vi "Robot Main.vi"() -> ()   [LabVIEW 2011]
doc: "This VI imlements the framework and scheduler for your robotics program. It should not be necessary to modify the framework. You are expected to add your code to the VIs called from Robot Main, the ones located in the Team Code within the project."
uses:
  GLOBALShooter.vi
panel:
  out "Timings":cluster{"Call Name":string, "Delta (ms)":u32}[](array[cluster])
  in  "Finish":bool
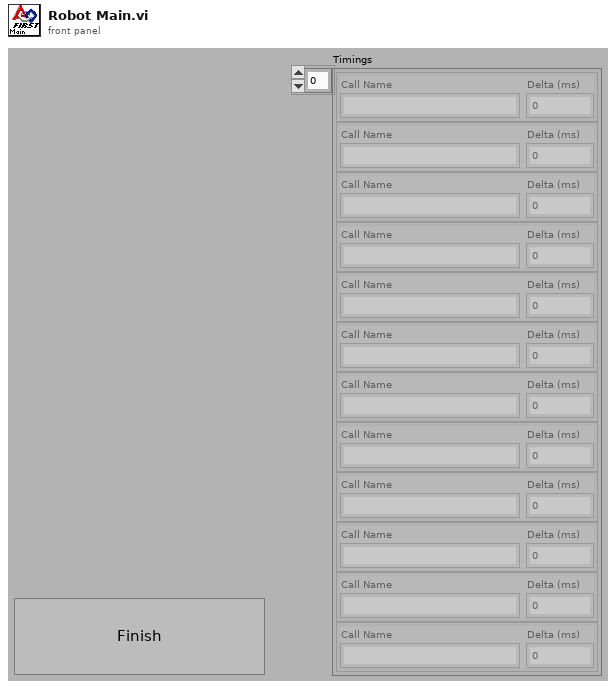
[diagram p1: front panel]
types:
  T1 = typedef "WPI_DriverStationMatch Info.ctl" = cluster{"Autonomous Elapsed Seconds":dbl, "TeleOp Elapsed Seconds":dbl, "Disabled Elapsed Seconds":dbl, "Visited Autonomous":bool, "Visited TeleOp":bool, "Visited Disabled":bool, "Autonomous Settings":cluster{"Autonomous Style":enum16{"Iterative", "Independent"}, "VI Refnum":refnum<vi>}}
  T2 = typedef "WPI_DriverStationDerivedRobotMode.ctl" = enum16{"Init", "Execute", "Stop"}
  T3 = typedef "WPI_DriverStationRobotMode.ctl" = enum16{"Autonomous Disabled", "Autonomous Enabled", "Teleop Disabled", "Teleop Enabled", "Timeout", "Finish"}
  T4 = typedef "WPI_GyroDevRef.ctl" = cluster{"DevStatus":errorcluster, "Analog Module":T5, "Analog Channel":T6, "Offset":dbl, "Gain (VoltsPerDegree/Second)":dbl}
  T5 = typedef "FPGA_TypedefAnalogModule.ctl" = enum16{"Analog Module 1", "Analog Module 2"}
  T6 = typedef "FPGA_AIChannel.ctl" = enum8{"AI 1", "AI 2", "AI 3", "AI 4", "AI 5", "AI 6", "AI 7", "AI 8", "Invalid"}
  T7 = typedef "WPI_EncoderDevRef.ctl" = cluster{"DevStatus":errorcluster, "EncoderIndex":T8, "CounterIndex":T9, "DistancePerCount":dbl, "Decoding Type":T10}
  T8 = typedef "FPGA_EncoderIdx.ctl" = enum8{"Enc 0", "Enc 1", "Enc 2", "Enc 3", "Invalid"}
  T9 = typedef "FPGA_CounterCtrSystemIndex.ctl" = enum8{"Ctr 0", "Ctr 1", "Ctr 2", "Ctr 3", "Ctr 4", "Ctr 5", "Ctr 6", "Ctr 7", "Invalid"}
  T10 = typedef "WPI_EncoderType.ctl" = enum16{"1x", "2x", "4x"}
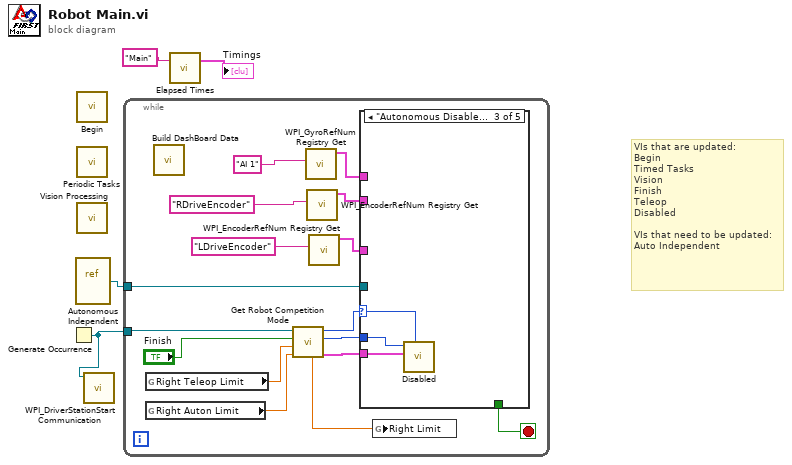
[diagram p0: block diagram]
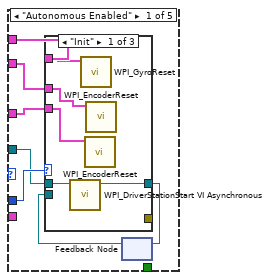
[diagram p2: hidden frame]
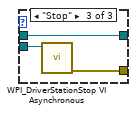
[diagram p4: hidden frame]
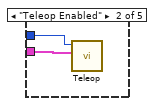
[diagram p5: hidden frame]
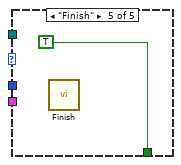
[diagram p7: hidden frame]
diagram:
  # "VIs that are updated:\nBegin\nTimed Tasks\nVision\nFinish\nTeleop\nDisabled\n\nVIs that need to be updated:\nAuto Independent"
  n1 = Generate Occurrence() -> (w4:refnum<k4>)
  n2 = vi-ref "Autonomous Independent.vi"() -> (w3:refnum<vi>)
  n3 = call "Begin.vi"() -> ()  [unwired: 1 in, 11 out]
  n4 = call "Periodic Tasks.vi"() -> ()  [unwired: 2 in, 10 out]
  n5 = call "Vision Processing.vi"() -> ()  [unwired: 1 in, 7 out]
  n6 = call <vilib>:"WPI_DriverStationStart Communication.vi"("occurrence"=w4) -> ()  [unwired: 11 out]
  n7 = while {
    tunnel: w4 -> [w18]
    tunnel: w3 -> [w14]
    stop <- w15 stop-if-true
    n8 = global read "GLOBALShooter.vi" "Right Teleop Limit"() -> (w6:dbl)
    n9 = global read "GLOBALShooter.vi" "Right Auton Limit"() -> (w5:dbl)
    n10 = call "Build DashBoard Data.vi"() -> ()  [unwired: 1 in, 11 out]
    n11 = call "Get Robot Competition Mode.vi"("Right Auton Limit"=w5, "Right Teleop Limit"=w6, "Finish"="Finish", "DS Occurrence"=w18) -> ("Match Info out"=w16:T1, "Call Context"=w20:T2, "Robot Mode"=w19:T3, "Right Limit"=w7:dbl)  [unwired: 4 out]
    n12 = call <vilib>:"WPI_GyroRefNum Registry Get.vi"("refnum name"="AI 1") -> ("GyroDevRef"=w13:T4)  [unwired: 9 in, 1 out]
    n13 = call <vilib>:"WPI_EncoderRefNum Registry Get.vi"("refnum name"="RDriveEncoder") -> ("EncoderDevRef"=w12:T7)  [unwired: 9 in, 1 out]
    n14 = call <vilib>:"WPI_EncoderRefNum Registry Get.vi"("refnum name"="LDriveEncoder") -> ("EncoderDevRef"=w11:T7)  [unwired: 9 in, 1 out]
    n15 = case shown="\"Autonomous Disabled\", \"Teleop Disabled\"" w19 {
      selector: w19 -> [_ _ w39 _ _]
      tunnel: w20 -> [w27 w38 w41 _ _]
      tunnel: w16 -> [_ w37 w40 _ _]
      tunnel: [_ _ _ _ TRUE] -> w15
      tunnel: w14 -> [w26 _ _ _ _]
      tunnel: w13 -> [w23 _ _ _ _]
      tunnel: w12 -> [w22 _ _ _ _]
      tunnel: w11 -> [w21 _ _ _ _]
      frame "Autonomous Enabled" {
        n16 = feedback #1() -> (w24:refnum<vi>)  [unwired: 1 out]
        n17 = case shown="\"Init\"" w27 {
          tunnel: w26 -> [w32 _ w35]
          tunnel: [w31 w33 w35] -> w25
          tunnel: w24 -> [_ w33 w36]
          tunnel: [_ _ w34] -> _
          tunnel: w23 -> [w30 _ _]
          tunnel: w22 -> [w29 _ _]
          tunnel: w21 -> [w28 _ _]
          frame "Init" {
            n18 = call <vilib>:"WPI_DriverStationStart VI Asynchronous.vi"("VI"=w32) -> ("VI out"=w31:refnum<vi>)  [unwired: 10 out]
            n19 = call <vilib>:"WPI_GyroReset.vi"("GyroDevRef"=w30) -> ()  [unwired: 9 in, 2 out]
            n20 = call <vilib>:"WPI_EncoderReset.vi"("EncoderDevRef"=w28) -> ()  [unwired: 9 in, 2 out]
            n21 = call <vilib>:"WPI_EncoderReset.vi"("EncoderDevRef"=w29) -> ()  [unwired: 9 in, 2 out]
          }
          frame "Execute", Default {
            # "Nothing to do"
          }
          frame "Stop" {
            n22 = call <vilib>:"WPI_DriverStationStop VI Asynchronous.vi"("VI Refnum"=w36) -> ("error out"=w34:errorcluster)  [unwired: 10 out]
          }
        }
        n23 = feedback-in #1(w25) -> ()
      }
      frame "Teleop Enabled" {
        n24 = call "Teleop.vi"("Match Info"=w37, "Call Context"=w38) -> ()  [unwired: 1 in, 9 out]
      }
      frame "Autonomous Disabled", "Teleop Disabled" {
        n25 = call "Disabled.vi"("Robot Mode"=w39, "Match Info"=w40, "Call Context"=w41) -> ()  [unwired: 1 in, 8 out]
      }
      frame "Timeout" {
      }
      frame "Finish" {
        n26 = call "Finish.vi"() -> ()  [unwired: 1 in, 7 out]
      }
    }
    n27 = global write "GLOBALShooter.vi" "Right Limit"(w7) -> ()
  }
  n28 = call "Elapsed Times.vi"("Call Name"="Main") -> ("Timings"=→"Timings":cluster{"Call Name":string, "Delta (ms)":u32}[])  [unwired: 2 in]
